vi "Write.vi"(0 "file path (UNC)":path, 1 "Text":string) -> ()   [LabVIEW 2018]
panel:
  out "concatenated string":string
  out "befor":string
  # "Probleme avec la liaison verte chelou"
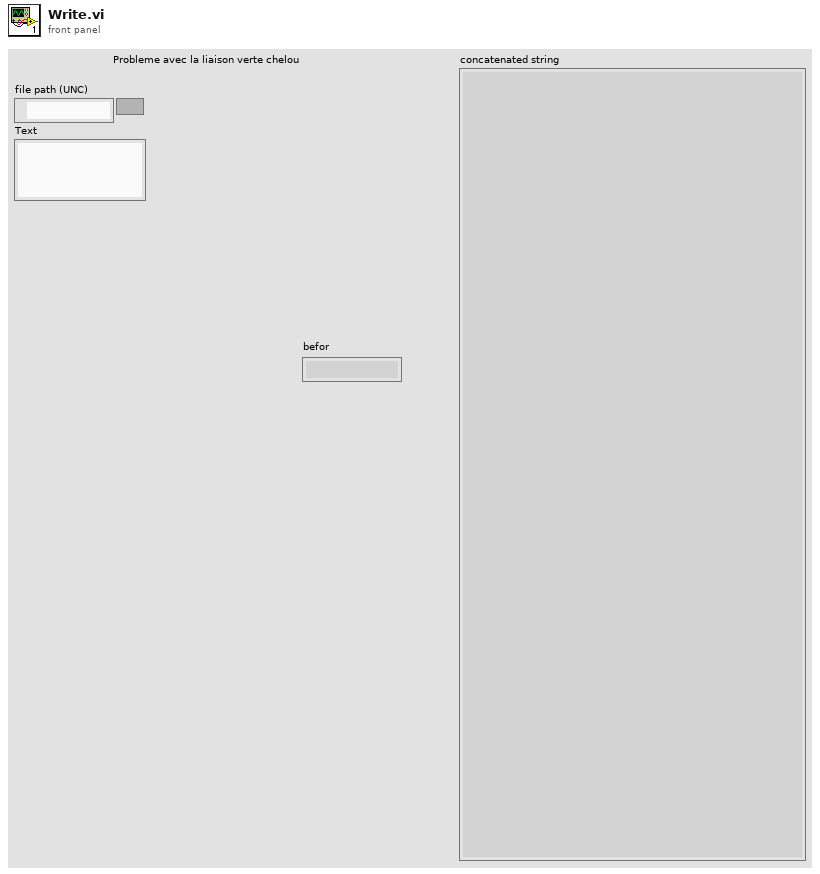
[diagram p1: front panel]
types:
  T1 = enum16{"open", "replace", "create", "open or create", "replace or create", "replace or create with confirmation"}
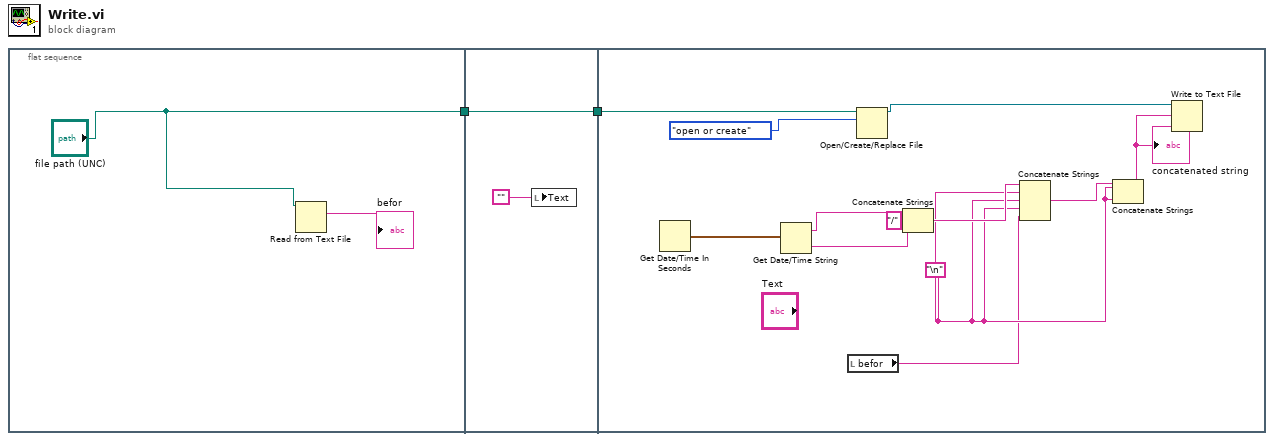
[diagram p0: block diagram]
diagram:
  n1 = flat-sequence {
    tunnel: ["file path (UNC)"] -> w1
    tunnel: [w5] -> w2
    tunnel: w1 -> [w5]
    tunnel: w2 -> [w9]
    frame #0 {
      n2 = Read from Text File(file (use dialog)="file path (UNC)") -> (text=→"befor":string)  [unwired: 3 in, 3 out]
    }
    frame #1 {
      n3 = local write "Text"("") -> ()
    }
    frame #2 {
      w8 = "\n"
      n4 = Get Date/Time In Seconds() -> (seconds since 1Jan1904=w16:timestamp)
      n5 = Get Date/Time String(seconds (now)=w16) -> (date string=w15:string, time string=w13:string)  [unwired: 2 in]
      n6 = local read "befor"() -> (w7:string)
      n7 = Open/Create/Replace File(file path (use dialog)=w9, operation (0:open)=T1."open or create") -> (refnum out=w18:refnum<file>)  [unwired: 4 in, 2 out]
      n8 = Concatenate Strings(w15, "/" ("string"), w13) -> (w14:string)
      n9 = Concatenate Strings(w14, w8, w8, w8, w7) -> (w11:string)
      n10 = Concatenate Strings(w11, w8, w8) -> (w10:string)
      "concatenated string" <- w10
      n11 = Write to Text File(file (use dialog)=w18, text=w10) -> ()  [unwired: 2 in, 3 out]
    }
  }
